vi "Set Bytes Progress by Ref.vi"(8 "error in (no error)":errorcluster, 10 "bytes downloaded":i64, 11 "HTTP GET Async ref in":refnum<data-value>) -> (0 "error out":errorcluster, 3 "HTTP GET Async ref out":refnum<data-value>)   [LabVIEW 2019, in "HTTP Client Extensions.lvlib" / "GET Async.lvclass"]
uses:
  GET Async.lvclass
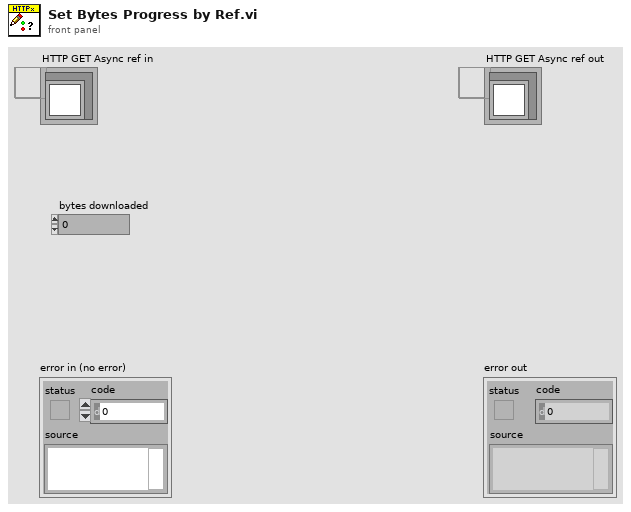
[diagram p1: front panel]
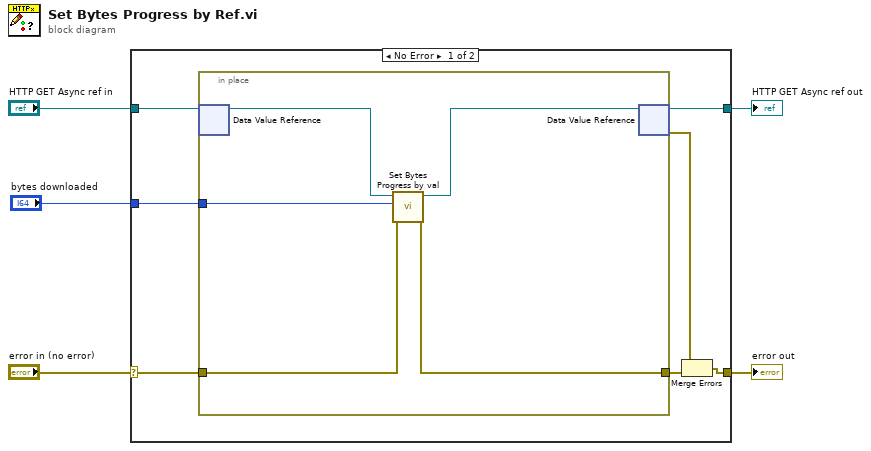
[diagram p0: block diagram]
diagram:
  n1 = case shown="No Error" "error in (no error)" {
    selector: "error in (no error)" -> [w10 w19]
    tunnel: [w7 w19] -> w4
    tunnel: [w8 w18] -> w2
    tunnel: "HTTP GET Async ref in" -> [w12 w18]
    tunnel: "bytes downloaded" -> [w11 _]
    frame No Error {
      n2 = in-place {
        in-place-border: w11 -> [w16]
        in-place-border: w10 -> [w15]
        in-place-border: [w14] -> w9
        n3 = in-place-dvr #1(w12) -> (w17:refnum<class "GET Async.lvclass">)  [unwired: 1 out]
        n4 = call "Set Bytes Progress by val.vi"("error in (no error)"=w15, "bytes downloaded"=w16, "HTTP GET Async in"=w17) -> ("error out"=w14:errorcluster, "HTTP GET Async out"=w13:refnum<class "GET Async.lvclass">)  [unwired: 7 in]
        n5 = in-place-dvr #1(w13) -> (w8:refnum<data-value>, w6:errorcluster)
      }
      n6 = Merge Errors(w6, w9) -> (w7:errorcluster)
    }
    frame Error {
    }
  }
  "error out" <- w4
  "HTTP GET Async ref out" <- w2
